vi "Is Server Stopped.vi"(7 "Server Alias":string, 8 "Error In":errorcluster) -> (0 "Error Out":errorcluster, 3 "Server Stopped":bool)   [LabVIEW 2013, in "TS.lvlib"]
doc: "This is an example of a dialog box for TestScript. The Python side can tell this dialog to run, asking for user input."
uses:
  TS.lvlib
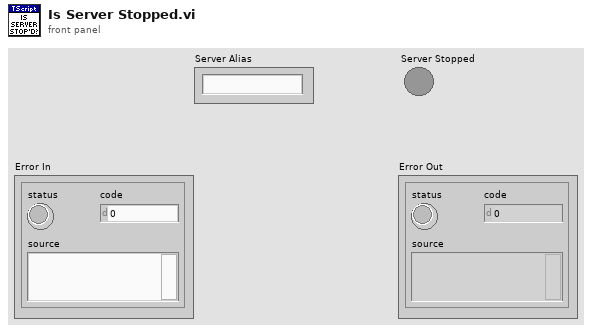
[diagram p1: front panel]
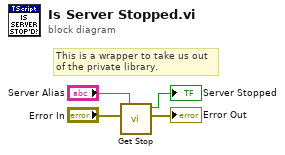
[diagram p0: block diagram]
diagram:
  # "This is a wrapper to take us out\nof the private library."
  n1 = call "Get Stop.vi"("Server Alias"="Server Alias", "Error In"="Error In") -> ("Error Out"=→"Error Out":errorcluster, "Stop"=→"Server Stopped":bool)  [unwired: 8 in]
